vi "c Spark Setpoint Command.vi"(5 "arbFFUnits":i32, 6 "arbFeedforward":sgl, 7 "pidSlot":i32, 8 "error in (no error)":errorcluster, 9 "ctrl":T1, 10 "value":sgl, 11 "handle":T2) -> (0 "error out":errorcluster, 2 "function return":T3, 3 "handle out":T2)   [LabVIEW 2023, in "REVLibDriver.lvlib"]
doc: "c_REVLib_ErrorCode c_Spark_SetpointCommand(c_Spark_handle handle, float value,\n c_Spark_ControlType ctrl,\n int pidSlot, float arbFeedforward,\n int arbFFUnits);"
uses:
  REVLibDriver.lvlib
  REVLibDriver.dll
  Custom Controls/c_Spark_handle.ctl
  subvi/RevLibError.ctl
  Custom Controls/c_Spark_ControlType.ctl
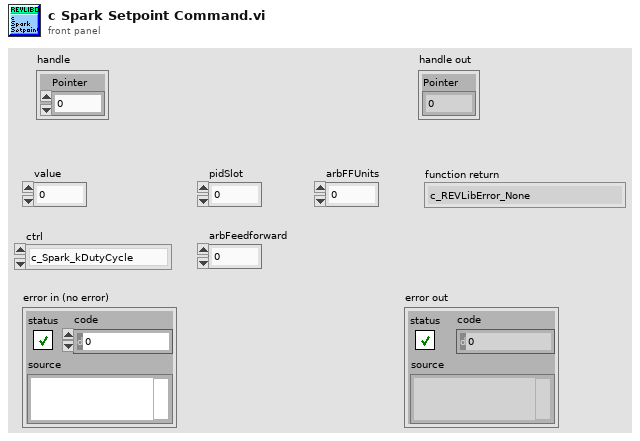
[diagram p1: front panel]
types:
  T1 = typedef "REVLibDriver.lvlib/c_Spark_ControlType.ctl" = enum16{"c_Spark_kDutyCycle", "c_Spark_kVelocity", "c_Spark_kVoltage", "c_Spark_kPosition", "c_Spark_kSmartMotion", "c_Spark_kCurrent", "c_Spark_kSmartVelocity", "c_Spark_kMAXMotion"}
  T2 = typedef "REVLibDriver.lvlib/c_Spark_handle.ctl" = cluster{"Pointer":u64}
  T3 = typedef "REVLibDriver.lvlib/RevLibError.ctl" = enum16{"c_REVLibError_None", "c_REVLibError_General", "c_REVLibError_CANTimeout", "c_REVLibError_NotImplemented", "c_REVLibError_HAL", "c_REVLibError_CantFindFirmware", "c_REVLibError_FirmwareTooOld", "c_REVLibError_FirmwareTooNew", "c_REVLibError_ParamInvalidID", "c_REVLibError_ParamMismatchType", "c_REVLibError_ParamAccessMode", "c_REVLibError_ParamInvalid", "c_REVLibError_ParamNotImplementedDeprecated", "c_REVLibError_FollowConfigMismatch", "c_REVLibError_Invalid", "c_REVLibError_SetpointOutOfRange", "c_REVLibError_Unknown", "c_REVLibError_CANDisconnected", "c_REVLibError_DuplicateCANId", "c_REVLibError_InvalidCANId", "c_REVLibError_SparkMaxDataPortAlreadyConfiguredDifferently", "c_REVLibError_SparkFlexBrushedWithoutDock", "c_REVLibError_InvalidBrushlessEncoderConfiguration", "c_REVLibError_FeedbackSensorIncompatibleWithDataPortConfig", "c_REVLibError_ParamInvalidChannel", "c_REVLibError_ParamInvalidValue", "c_REVLibError_CannotPersistParametersWhileEnabled", "c_REVLibError_NotReadyToReceiveCommand", "c_REVLibError_NumCodes"}
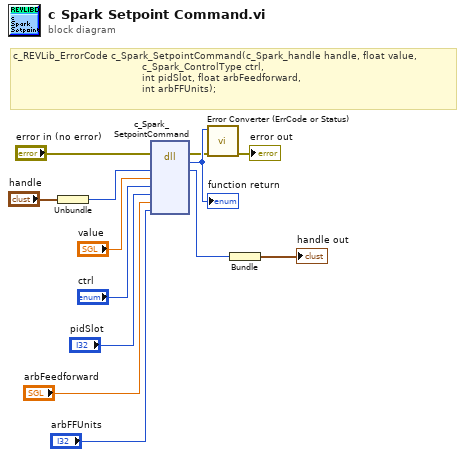
[diagram p0: block diagram]
diagram:
  # "c_REVLib_ErrorCode c_Spark_SetpointCommand(c_Spark_handle handle, float value,\n                                           c_Spark_ControlType ctrl,\n                                           int pidSlot, float arbFeedforward,\n                                           int arbFFUnits);"
  n1 = Unbundle("handle") -> ("Pointer"=w2:u64)
  n2 = dll-call lib="REVLibDriver.*" fn="c_Spark_SetpointCommand"(error in="error in (no error)", "handle"=w2, "value"="value", "ctrl"="ctrl", "pidSlot"="pidSlot", "arbFeedforward"="arbFeedforward", "arbFFUnits"="arbFFUnits") -> (error out=w4:errorcluster, "return type"=w13:u32, "handle"=w11:u64)  [unwired: 7 in, 1 out]
  "function return" <- w13
  n3 = call "Error Converter (ErrCode or Status).vi"("error in (no error)"=w4, "error code"=w13) -> ("error out"=→"error out":errorcluster)  [unwired: 9 in]
  n4 = Bundle("handle"=w11) -> (→"handle out":cluster{"handle":u64})  [unwired: 1 in]
